vi "Publish I16.vi"(8 "error in (no error)":errorcluster, 10 "I16":i16, 11 "MVC Subscription in":refnum<class "MVC Subscription.lvclass">) -> (0 "error out":errorcluster, 3 "MVC Subscription out":refnum<class "MVC Subscription.lvclass">)   [LabVIEW 2014, in "MVC Subscription.lvlib" / "MVC Subscription.lvclass"]
uses:
  MVC Subscription.lvclass
  MVC Subscription.lvclass/MVC Subscription.ctl
  Messages/Message (I16)/_Message (I16).lvclass
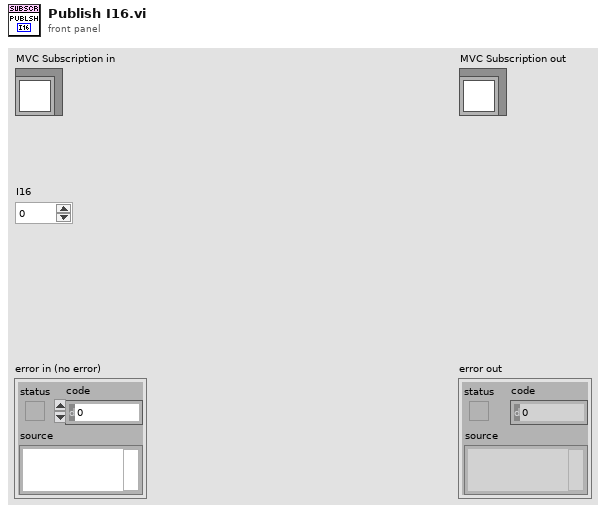
[diagram p1: front panel]
types:
  T1 = typedef "MVC Subscription.lvlib/MVC Subscription.lvclass/Cluster - Individual Subscription.ctl" = cluster{"Enqueuer":refnum<class "Message Enqueuer.lvclass">, "Message":refnum<class "Message.lvclass">}
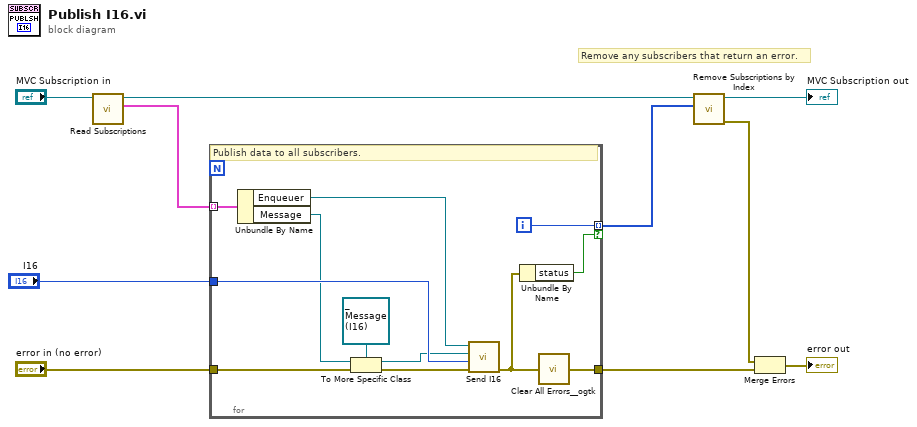
[diagram p0: block diagram]
diagram:
  # "Remove any subscribers that return an error."
  n1 = call "Read Subscriptions.vi"("MVC Subscription in"="MVC Subscription in") -> ("Subscriptions"=w5:T1[], "MVC Subscription out"=w8:refnum<class "MVC Subscription.lvclass">)  [unwired: 9 in]
  n2 = for {
    tunnel: "I16" -> [w21]
    tunnel: w5 -> [w20] mode=indexing
    tunnel: "error in (no error)" -> [w22]
    tunnel: [w13] -> w1
    tunnel: [w12] -> w6 mode=indexing if=w11
    i -> [w12]
    # "Publish data to all subscribers."
    n3 = Unbundle By Name(w20) -> ("Enqueuer"=w19:refnum<class "Message Enqueuer.lvclass">, "Message"=w17:refnum<class "Message.lvclass">)
    n4 = To More Specific Class(target class=refnum<class "_Message (I16).lvclass"> refnum ("_Message (I32).lvclass"), reference=w17, error in=w22) -> (specific class reference=w15:refnum<class "_Message (I16).lvclass">, error out=w18:errorcluster)
    n5 = call-dynamic "Send I16.vi"("error in"=w18, "I16"=w21, "_Message (I16) in"=w15, "Enqueuer"=w19) -> ("error out"=w14:errorcluster)  [unwired: 6 in, 1 out]
    n6 = Unbundle By Name(w14) -> ("status"=w11:bool)
    n7 = call <userlib>:"Clear All Errors__ogtk.vi"("Error In"=w14) -> ("Error Out"=w13:errorcluster)  [unwired: 3 in]
  }
  n8 = call "Remove Subscriptions by Index.vi"("Index of Elements to Remove"=w6, "MVC Subscription in"=w8) -> ("error out"=w2:errorcluster, "MVC Subscription out"=→"MVC Subscription out":refnum<class "MVC Subscription.lvclass">)  [unwired: 8 in]
  n9 = Merge Errors(w2, w1) -> (→"error out":errorcluster)
